vi "TDMS Upload Example.vi"() -> ()   [LabVIEW 2024]
doc: "TDMS upload example."
uses:
  Sift API/Sift Client.lvclass
panel:
  in  "API gRPC URL":string
  in  "Run Name":string="TDMS Upload Example"
  in  "Asset Name":string="LabVIEW-TDMS-Example"
  in  "Absolute Filepath":path
  out "Error":errorcluster
  in  "API Key":string
  in  "API REST URL":string
  # "Sift TDMS Upload Example (Waveform)"
  # "Run this example to test uploading TDMS files to Sift. The channels\nin this example are Waveform channels."
  # "Instructions\n\n1. Fill in the API  URLs and API Key. Visit this URL for more information on authentication\n    https://docs.siftstack.com/docs/api/authentication\n\n2. Select a TDMS file to upload. There is a \"sample_data.tdms\" file in the same Example directory of this VI.\n\n3. Run the VI.\n\n3. The VI should run to completetion with no errors. Navigate to the Sift home page and find the \n     Run to see the example data."
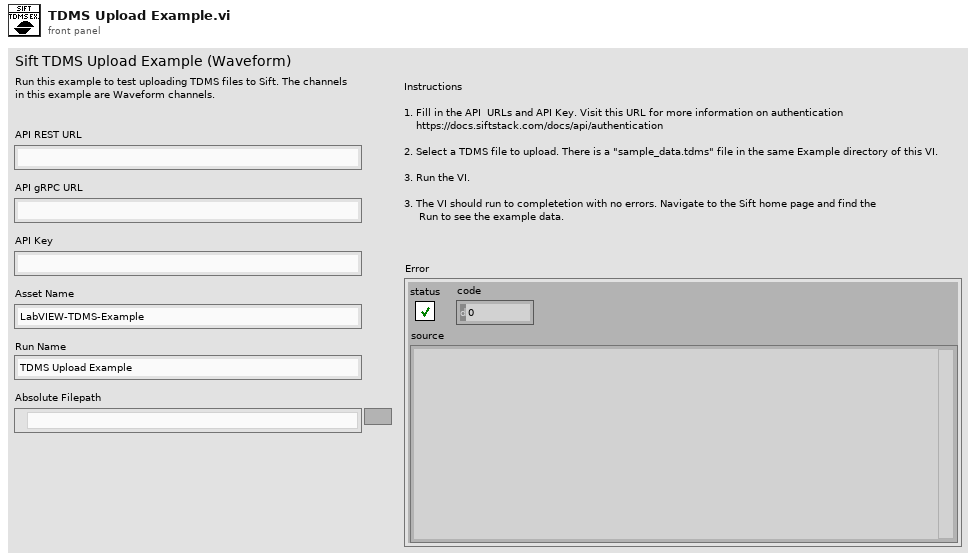
[diagram p1: front panel]
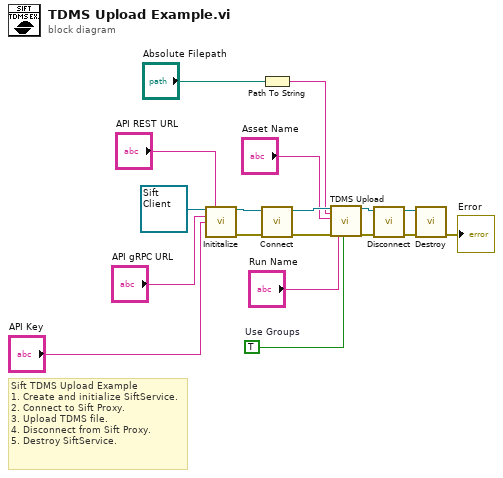
[diagram p0: block diagram]
diagram:
  w3 = TRUE  # Use Groups
  # "Sift TDMS Upload Example\n1. Create and initialize SiftService.\n2. Connect to Sift Proxy.\n3. Upload TDMS file.\n4. Disconnect from Sift Proxy.\n5. Destroy SiftService."
  n1 = call-dynamic "Inititalize.vi"("Sift Client in"=refnum<class "Sift Client.lvclass"> refnum ("Sift Client.lvlib:Sift Client.lvclass"), "REST URL"="API REST URL", "GRPC URL"="API gRPC URL", "API Key"="API Key") -> ("Sift Client out"=w15:refnum<class "Sift Client.lvclass">, "error out"=w14:errorcluster)  [unwired: 10 in]
  n2 = Path To String(path="Absolute Filepath") -> (string=w5:string)
  n3 = call-dynamic "Connect.vi"("error in (no error)"=w14, "Sift Client in"=w15) -> ("error out"=w12:errorcluster, "Sift Client out"=w13:refnum<class "Sift Client.lvclass">)  [unwired: 7 in, 1 out]
  n4 = call-dynamic "TDMS Upload.vi"("Sift Client in"=w13, "Filepath"=w5, "Asset Name"="Asset Name", "error in (no error)"=w12, "Run Name"="Run Name", "Group Into Components"=w3) -> ("Sift Client out"=w11:refnum<class "Sift Client.lvclass">, "error out"=w10:errorcluster)  [unwired: 12 in]
  n5 = call-dynamic "Disconnect.vi"("error in (no error)"=w10, "Sift Client in"=w11) -> ("error out"=w8:errorcluster, "Sift Client out"=w9:refnum<class "Sift Client.lvclass">)  [unwired: 8 in]
  n6 = call-dynamic "Destroy.vi"("error in (no error)"=w8, "Sift Client in"=w9) -> ("error out"=→"Error":errorcluster)  [unwired: 8 in, 1 out]
